vi "read_cooling_P.vi"(8 "error in (no error)":errorcluster, 11 "VISA resource name":refnum<visa-resource-name>) -> (0 "error out":errorcluster, 1 "Unit":string, 2 "P":dbl, 3 "VISA resource name out":refnum<visa-resource-name>)   [LabVIEW 2018]
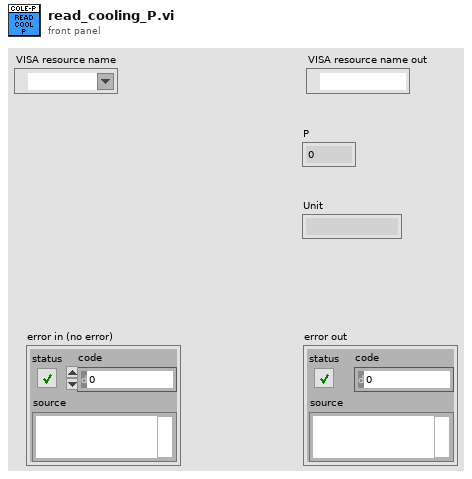
[diagram p1: front panel]
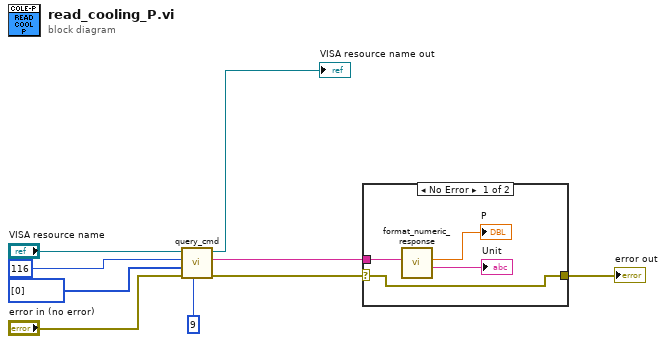
[diagram p0: block diagram]
diagram:
  n1 = call "query_cmd.vi"("Number of bytes in response"=u32 9, "error in (no error)"="error in (no error)", "Data bytes"=u8[] [0], "Command byte"=u8 116, "VISA resource name"="VISA resource name") -> ("error out"=w2:errorcluster, "Response"=w3:string, "VISA resource name out"=→"VISA resource name out":refnum<visa-resource-name>)  [unwired: 4 in]
  n2 = case shown="No Error" w2 {
    selector: w2 -> [w10 w14]
    tunnel: w3 -> [w13 _]
    tunnel: [w10 w14] -> w1
    frame No Error {
      n3 = call "format_numeric_response.vi"("Response"=w13) -> ("Unit"=→"Unit":string, "Value"=→"P":dbl)  [unwired: 9 in]
    }
    frame Error {
    }
  }
  "error out" <- w1
